vi "FRIC_navX_Internal_ProcessingLoop_UpdateAE.vi"() -> (1 "Board Information":T11 {"Board"."Hardware Revision" items=["navX-MXP"=33, "navX-Micro"=40]; "Omnimount Config" items=["DEFAULT", "X_UP", "X_DOWN", "Y_UP", "Y_DOWN", "Z_UP", "Z_DOWN"]}, 2 "MPUTemp":dbl, 3 "Displacement":T12, 4 "Linear Acceleration":T8, 6 "Offsets":T7, 8 "Quaternion":T5, 10 "YRPHfH":T1, 12 "Raw Values (out)":T6, 13 "Status":T4 {"OP Status" items=["INITIALIZING", "SELFTEST_IN_PROGRESS", "ERROR", "IMU_AUTOCAL_IN_PROGRESS", "NORMAL"]; "Calibration Status" items=["IMU_CAL_STATE_MASK"=3, "IMU_CAL_STATE_INPROGRESS"=0, "IMU_CAL_STATE_ACCUMULATE"=1, "IMU_CAL_STATE_COMPLETE"=2]}, 14 "Timestamp":u32)   [LabVIEW 2015, in "navX AE v1.lvlib"]
uses:
  navX AE v1.lvlib
  navX Library v2/_TypeDefs/Flags/Z900_navX_Flags_HardwareRevTypeDef.ctl
  navX Library v2/_TypeDefs/Flags/Z900_navX_Flags_OmnimountConfigTypeDef.ctl
  navX Library v2/_TypeDefs/Flags/Z900_navX_Flags_OpStatusTypeDef.ctl
  navX Library v2/_TypeDefs/Flags/Z900_navX_Flags_CalibrationStatusTypeDef.ctl
  navX Library v2/navX Library v2.lvlib
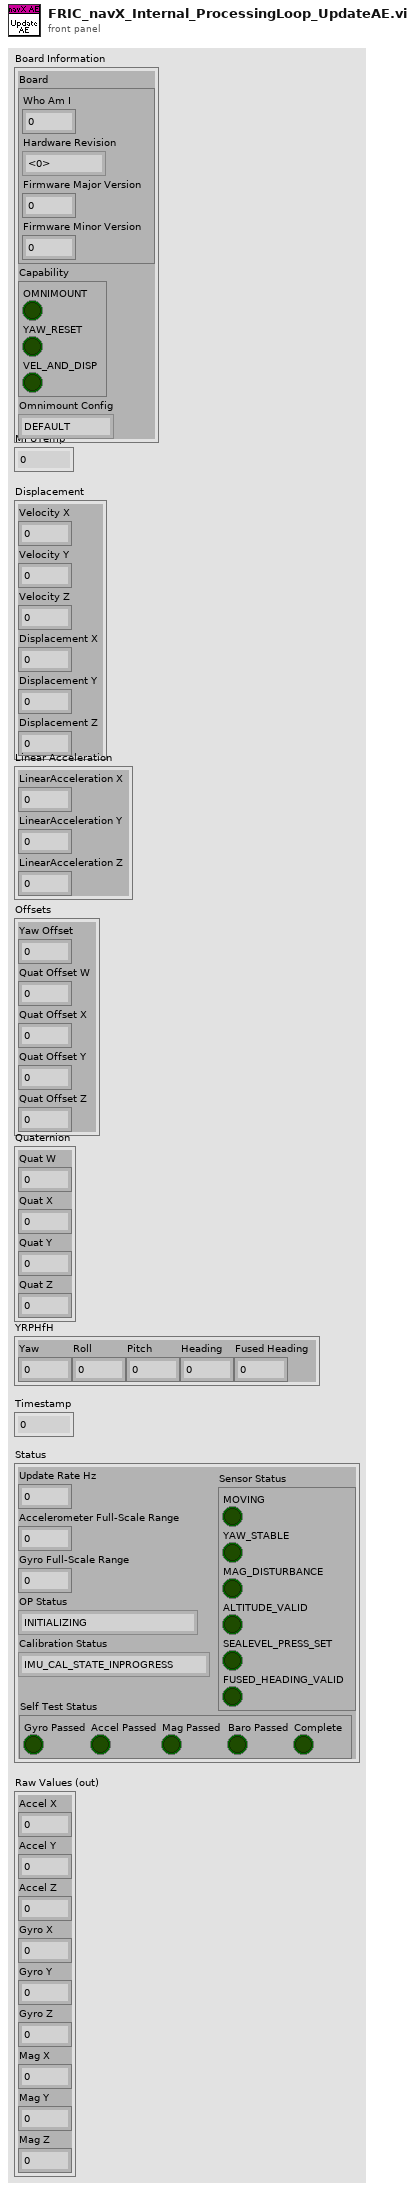
[diagram p1: front panel]
types:
  T1 = cluster{"Yaw":dbl, "Roll":dbl, "Pitch":dbl, "Heading":dbl, "Fused Heading":dbl}
  T2 = typedef "navX Library v2.lvlib/Z900_navX_Flags_OpStatusTypeDef.ctl" = u8
  T3 = typedef "navX Library v2.lvlib/Z900_navX_Flags_CalibrationStatusTypeDef.ctl" = u8
  T4 = cluster{"Update Rate Hz":u8, "Accelerometer Full-Scale Range":u8, "Gyro Full-Scale Range":u16, "OP Status":T2, "Calibration Status":T3, "Sensor Status":cluster{"MOVING":bool, "YAW_STABLE":bool, "MAG_DISTURBANCE":bool, "ALTITUDE_VALID":bool, "SEALEVEL_PRESS_SET":bool, "FUSED_HEADING_VALID":bool}, "Self Test Status":cluster{"Gyro Passed":bool, "Accel Passed":bool, "Mag Passed":bool, "Baro Passed":bool, "Complete":bool}}
  T5 = cluster{"Quat W":dbl, "Quat X":dbl, "Quat Y":dbl, "Quat Z":dbl}
  T6 = cluster{"Accel X":dbl, "Accel Y":dbl, "Accel Z":dbl, "Gyro X":dbl, "Gyro Y":dbl, "Gyro Z":dbl, "Mag X":dbl, "Mag Y":dbl, "Mag Z":dbl}
  T7 = cluster{"Yaw Offset":dbl, "Quat Offset W":dbl, "Quat Offset X":dbl, "Quat Offset Y":dbl, "Quat Offset Z":dbl}
  T8 = cluster{"LinearAcceleration X":dbl, "LinearAcceleration Y":dbl, "LinearAcceleration Z":dbl}
  T9 = typedef "navX Library v2.lvlib/Z900_navX_Flags_HardwareRevTypeDef.ctl" = u8
  T10 = typedef "navX Library v2.lvlib/Z900_navX_Flags_OmnimountConfigTypeDef.ctl" = u8
  T11 = cluster{"Board":cluster{"Who Am I":u8, "Hardware Revision":T9, "Firmware Major Version":u8, "Firmware Minor Version":u8}, "Capability":cluster{"OMNIMOUNT":bool, "YAW_RESET":bool, "VEL_AND_DISP":bool}, "Omnimount Config":T10}
  T12 = cluster{"Velocity X":dbl, "Velocity Y":dbl, "Velocity Z":dbl, "Displacement X":dbl, "Displacement Y":dbl, "Displacement Z":dbl}
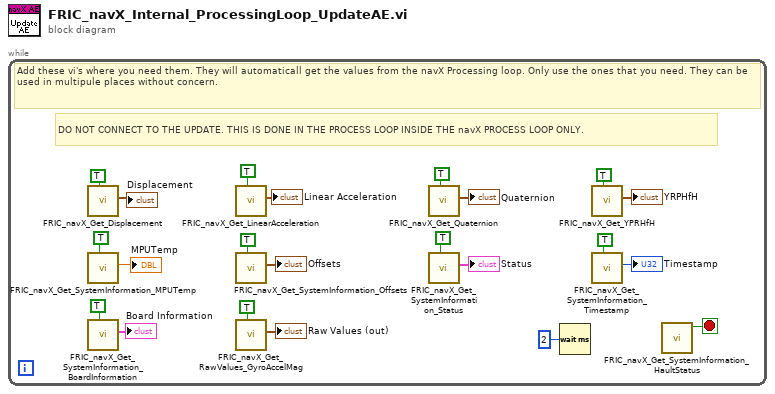
[diagram p0: block diagram]
diagram:
  n1 = while {
    stop <- w1 stop-if-true
    # "DO NOT CONNECT TO THE UPDATE. THIS IS DONE IN THE PROCESS LOOP INSIDE THE navX PROCESS LOOP ONLY."
    # "Add these vi's where you need them. They will automaticall get the values from the navX Processing loop. Only use the ones that you need. They can be used in multipule places without concern."
    n2 = call "FRIC_navX_Get_Displacement.vi"("Update"=TRUE) -> ("Displacement"=→"Displacement":T12)  [unwired: 10 in]
    n3 = call "FRIC_navX_Get_SystemInformation_MPUTemp.vi"("Update"=TRUE) -> ("MPUTemp"=→"MPUTemp":dbl)  [unwired: 10 in]
    n4 = call "FRIC_navX_Get_SystemInformation_BoardInformation.vi"("Update"=TRUE) -> ("Board Information"=→"Board Information":T11)  [unwired: 10 in]
    n5 = call "FRIC_navX_Get_LinearAcceleration.vi"("Update"=TRUE) -> ("Linear Acceleration"=→"Linear Acceleration":T8)  [unwired: 10 in]
    n6 = call "FRIC_navX_Get_SystemInformation_Offsets.vi"("Update"=TRUE) -> ("Offsets"=→"Offsets":T7)  [unwired: 10 in]
    n7 = call "FRIC_navX_Get_RawValues_GyroAccelMag.vi"("Update"=TRUE) -> ("Raw Values (out)"=→"Raw Values (out)":T6)  [unwired: 10 in]
    n8 = call "FRIC_navX_Get_Quaternion.vi"("Update"=TRUE) -> ("Quaternion"=→"Quaternion":T5)  [unwired: 10 in]
    n9 = call "FRIC_navX_Get_SystemInformation_Status.vi"("Update"=TRUE) -> ("Status"=→"Status":T4)  [unwired: 10 in]
    n10 = Wait (ms)(milliseconds to wait=u32 2) -> ()  [unwired: 1 out]
    n11 = call "FRIC_navX_Get_YPRHfH.vi"("Update"=TRUE) -> ("YRPHfH"=→"YRPHfH":T1)  [unwired: 10 in]
    n12 = call "FRIC_navX_Get_SystemInformation_Timestamp.vi"("Update"=TRUE) -> ("Timestamp"=→"Timestamp":u32)  [unwired: 10 in]
    n13 = call "FRIC_navX_Get_SystemInformation_HaultStatus.vi"() -> ("Hault"=w1:bool)  [unwired: 11 in]
  }
